vi "From JSON Text.vi"(7 "Data Type and Default Value":variant, 9 "error in":errorcluster, 10 "Offset":i32, 11 "JSON":string) -> (1 "error out":errorcluster, 3 "Data out":variant)   [LabVIEW 2021, in "jsontext.facade.lvlib"]
doc: "Convert JSON to the LabVIEW Data Type entered."
uses:
  jsontext.facade.lvlib
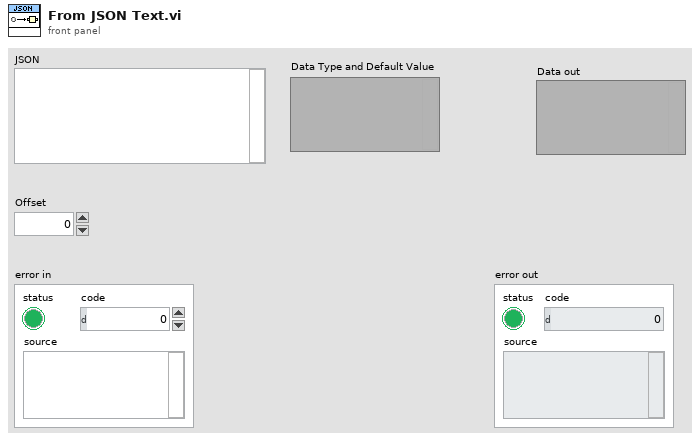
[diagram p1: front panel]
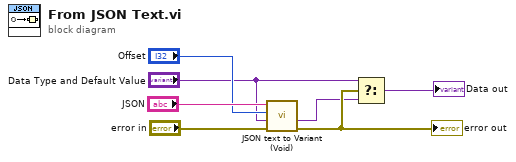
[diagram p0: block diagram]
diagram:
  n1 = call "JSON text to Variant (Void).vi"("error in (no error)"="error in", "Data Type"="Data Type and Default Value", "Offset"="Offset", "JSON"="JSON") -> ("error out"=w4:errorcluster, "Variant out"=w1:variant)  [unwired: 6 in]
  "error out" <- w4
  n2 = Select(t="Data Type and Default Value", s=w4, f=w1) -> (s? t:f=→"Data out":variant)
